vi "ремонт Кластеры-01-порядок.vi"() -> ()   [LabVIEW 2017]
panel:
  out "Cluster 2":T1
  in  "Cluster":T1
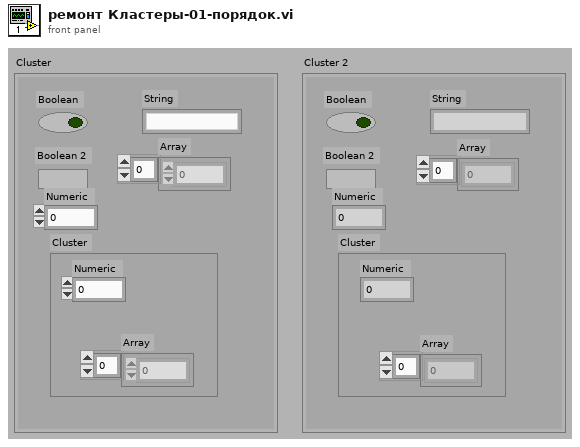
[diagram p1: front panel]
types:
  T1 = cluster{"Boolean":bool, "String":string, "Boolean 2":bool, "Array":dbl[], "Numeric":dbl, "Cluster":cluster{"Numeric":i32, "Array":u8[]}}
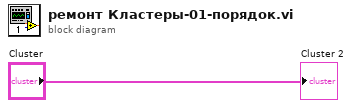
[diagram p0: block diagram]
diagram:
  "Cluster 2" <- "Cluster"
